vi "Instances set user string.vi"(1 "Dates undelivered in":timestamp[](array[timestamp]), 2 "Dates in":timestamp[](array[timestamp])) -> (0 "User string":string)   [LabVIEW 2015]
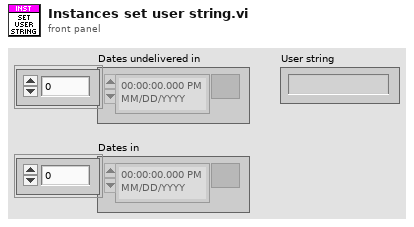
[diagram p1: front panel]
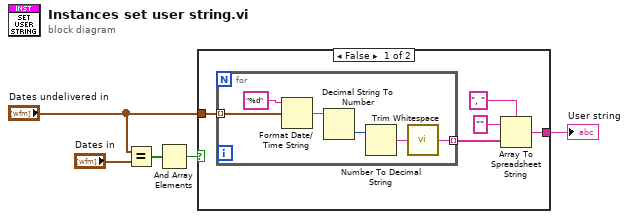
[diagram p0: block diagram]
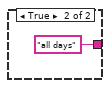
[diagram p2: hidden frame]
diagram:
  n1 = Equal?(x="Dates undelivered in", y="Dates in") -> (x = y?=w2:bool[])
  n2 = And Array Elements(Boolean array=w2) -> (logical AND=w3:bool)
  n3 = case shown="False" w3 {
    tunnel: [w7 "all days"] -> w5
    tunnel: "Dates undelivered in" -> [w10 _]
    frame False {
      n4 = for {
        tunnel: w10 -> [w16] mode=indexing
        tunnel: [w11] -> w9 mode=indexing
        n5 = Format Date/Time String(time format string (%c)="%d", seconds (now)=w16) -> (date/time string=w12:string)  [unwired: 1 in]
        n6 = Decimal String To Number(string=w12) -> (number=w14:i32)  [unwired: 2 in, 1 out]
        n7 = Number To Decimal String(number=w14) -> (decimal integer string=w13:string)  [unwired: 1 in]
        n8 = call <vilib>:"Trim Whitespace.vi"("string"=w13) -> ("trimmed string"=w11:string)  [unwired: 1 in]
      }
      n9 = Array To Spreadsheet String(delimiter (Tab)=", ", array=w9, 3:"" ("format string")) -> (spreadsheet string=w7:string)
    }
    frame True {
    }
  }
  "User string" <- w5
